vi "Add Legend.vi"(8 "error in (no error)":errorcluster, 10 ".NET MSChart Legend":refnum<k24>, 11 ".NET MSChart":refnum<k24>) -> (0 "error out":errorcluster)   [LabVIEW 2015, in "Graph Extensions MSChart.lvlib"]
uses:
  Graph Extensions MSChart.lvlib
  System.Windows.Forms.DataVisualization
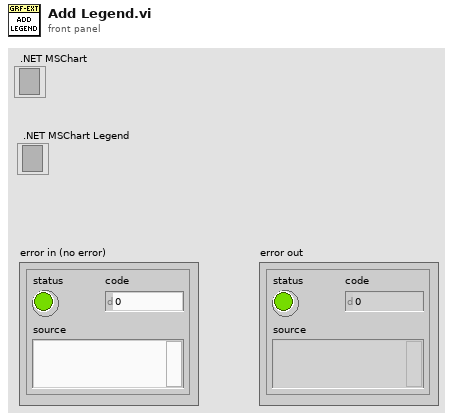
[diagram p1: front panel]
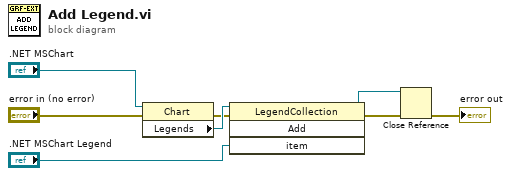
[diagram p0: block diagram]
diagram:
  n1 = property class="Chart"(reference=".NET MSChart", error in="error in (no error)") -> (error out=w5:errorcluster, "Legends"=w6:refnum<k24>)  [unwired: 1 out]
  n2 = invoke class="LegendCollection" method="Add"(reference=w6, error in=w5, "item"=".NET MSChart Legend") -> (reference out=w1:refnum<k24>, error out=w4:errorcluster)  [unwired: 1 in, 2 out]
  n3 = Close Reference(reference=w1, error in (no error)=w4) -> (error out=→"error out":errorcluster)
